vi "RTS Asyncrouns Write Setup.vi"(6 "Data":dbl[][](array[numeric]), 7 "Log System Time?":bool=TRUE, 8 "error in (no error)":errorcluster, 9 "Headers":string[](array[string]), 10 "Group Name":string, 11 "Refnum in":refnum<k34>) -> (0 "error out":errorcluster, 3 "Refnum out":refnum<k34>)   [LabVIEW 2016]
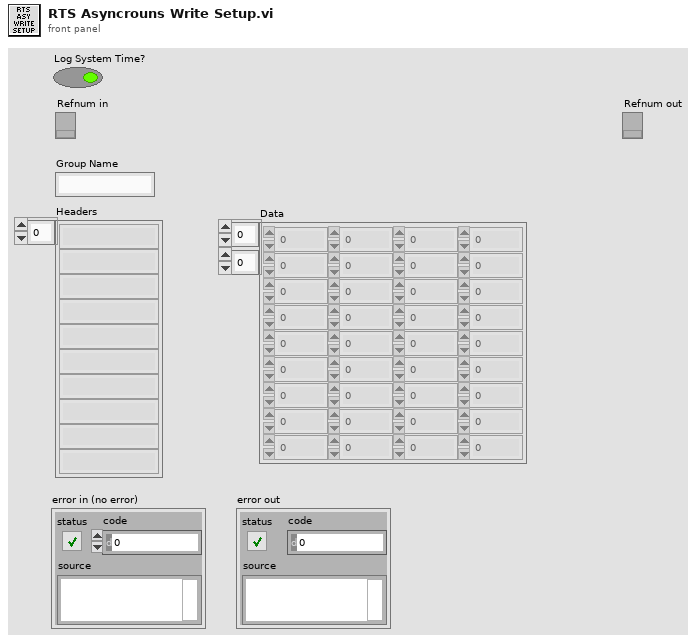
[diagram p1: front panel]
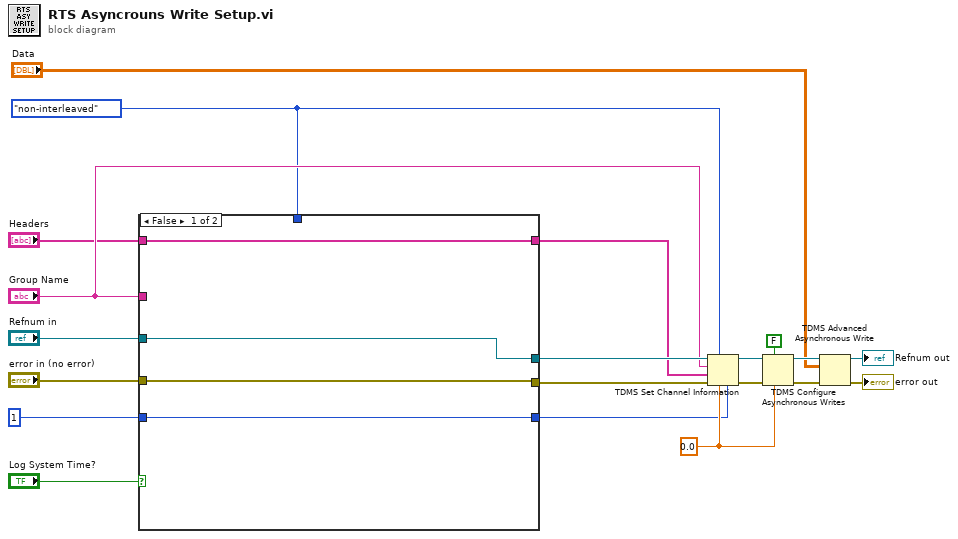
[diagram p0: block diagram]
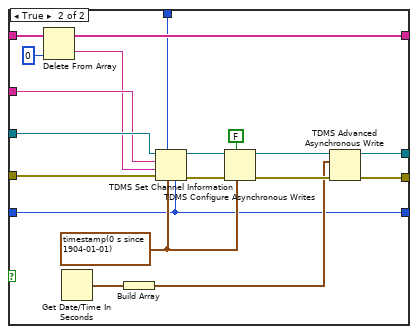
[diagram p2: hidden frame]
diagram:
  w4 = enum16{"non-interleaved", "interleaved"}."non-interleaved" ("data layout (0:non-interleaved)")
  w13 = 0.0 ("data type")
  n1 = case shown="False" "Log System Time?" {
    tunnel: "error in (no error)" -> [w22 w38]
    tunnel: [w22 w37] -> w10
    tunnel: "Refnum in" -> [w21 w36]
    tunnel: [w21 w33] -> w8
    tunnel: "Group Name" -> [_ w32]
    tunnel: "Headers" -> [w24 w31]
    tunnel: [w24 w28] -> w5
    tunnel: w4 -> [_ w27]
    tunnel: u32 1 ("samples per channel") -> [w23 w25]
    tunnel: [w23 w25] -> w1
    frame False {
    }
    frame True {
      w41 = timestamp(0 s since 1904-01-01)
      n2 = Delete From Array(array=w31, index=0) -> (deleted portion=w29:string, array with subset deleted=w28:string[])  [unwired: 1 in]
      n3 = Get Date/Time In Seconds() -> (seconds since 1Jan1904=w40:timestamp)
      n4 = Build Array(w40) -> (w39:timestamp[])
      n5 = TDMS Set Channel Information(4:w25, 6:w41, 7:w27, 8:w38, 9:w29, 10:w32, 11:w36) -> (0:w42:errorcluster, 3:w35:refnum<k34>)
      n6 = TDMS Configure Asynchronous Writes(6:w41, 7:FALSE ("pre-allocate? (F)"), 8:w42, 11:w35) -> (0:w43:errorcluster, 3:w34:refnum<k34>)  [unwired: 3 in]
      n7 = TDMS Advanced Asynchronous Write(8:w43, 10:w39, 11:w34) -> (0:w37:errorcluster, 3:w33:refnum<k34>)
    }
  }
  n8 = TDMS Set Channel Information(4:w1, 6:w13, 7:w4, 8:w10, 9:w5, 10:"Group Name", 11:w8) -> (0:w18:errorcluster, 3:w19:refnum<k34>)
  n9 = TDMS Configure Asynchronous Writes(6:w13, 7:FALSE ("pre-allocate? (F)"), 8:w18, 11:w19) -> (0:w16:errorcluster, 3:w17:refnum<k34>)  [unwired: 3 in]
  n10 = TDMS Advanced Asynchronous Write(8:w16, 10:"Data", 11:w17) -> (0:→"error out":errorcluster, 3:→"Refnum out":refnum<k34>)
